vi "Config Alarm.vi"(0 "VISA resource name":refnum<visa-resource-name>, 1 "Alarm (F: Alarm Disabled)":bool, 2 "Beeper (F: Beeper Disabled)":bool, 3 "Latching (F: Alarm Latch OFF)":bool, 5 "Input (1)":dbl=1.0 min=1.0 max=8.0 step=1.0, 9 "Alarm Source (0:Kelvin)":u16(ring) items=["Kelvin", "Celsius", "Sensor Units", "Linear Data"], 11 "error in (no error)":errorcluster, 12 "High Value (0.0000)":dbl min=-9999.9 max=9999.9 step=0.0001 format="%.4f", 13 "Deadband (0.0000)":dbl min=0.0 max=9999.9 step=0.0001 format="%.4f", 14 "Low Value (0.0000)":dbl min=-9999.9 max=9999.9 step=0.0001 format="%.4f") -> (4 "VISA resource name out":refnum<visa-resource-name>, 15 "error out":errorcluster)   [LabVIEW 2012, in "Lake Shore Cryotronics 218.lvlib"]
doc: "This VI configures all alarm functions for the selected input. Alarm functions include source, on/off, high value, low value, deadband, and latching parameters. This VI also enables/disables the system beeper, this control applies to all inputs."
uses:
  <instrlib>/Lake Shore Cryotronics 218/Lake Shore Cryotronics 218.lvlib
panel:
  # "Alarm Enabled"
  # "Alarm Latch ON"
  # "Alarm Disabled"
  # "Alarm Latch OFF"
  # "Beeper Enabled"
  # "Beeper Disabled"
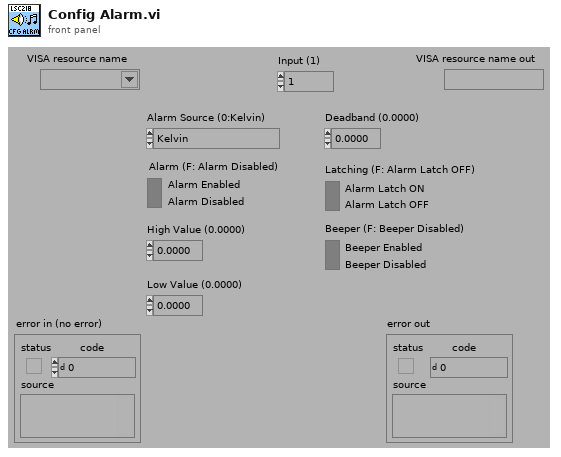
[diagram p1: front panel]
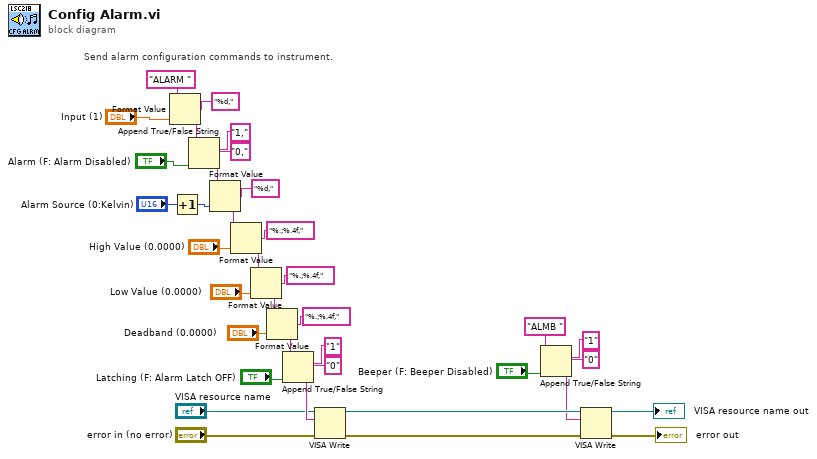
[diagram p0: block diagram]
diagram:
  # "Send alarm configuration commands to instrument."
  n1 = Format Value(string ("")="ALARM ", format string="%d,", value (0)="Input (1)") -> (output string=w21:string)
  n2 = Increment(x="Alarm Source (0:Kelvin)") -> (x+1=w23:u16)
  n3 = Append True/False String(1:"Alarm (F: Alarm Disabled)", 2:"0,", 3:"1,", 4:w21) -> (0:w20:string)
  n4 = Format Value(string ("")=w20, format string="%d,", value (0)=w23) -> (output string=w19:string)
  n5 = Format Value(string ("")=w19, format string="%.;%.4f,", value (0)="High Value (0.0000)") -> (output string=w18:string)
  n6 = Format Value(string ("")=w18, format string="%.;%.4f,", value (0)="Low Value (0.0000)") -> (output string=w16:string)
  n7 = Format Value(string ("")=w16, format string="%.;%.4f,", value (0)="Deadband (0.0000)") -> (output string=w11:string)
  n8 = Append True/False String(1:"Latching (F: Alarm Latch OFF)", 2:"0", 3:"1", 4:w11) -> (0:w10:string)
  n9 = VISA Write(VISA resource name="VISA resource name", write buffer=w10, error in (no error)="error in (no error)") -> (VISA resource name out=w32:refnum<visa-resource-name>, error out=w31:errorcluster)  [unwired: 1 out]
  n10 = Append True/False String(1:"Beeper (F: Beeper Disabled)", 2:"0", 3:"1", 4:"ALMB ") -> (0:w7:string)
  n11 = VISA Write(VISA resource name=w32, write buffer=w7, error in (no error)=w31) -> (VISA resource name out=→"VISA resource name out":refnum<visa-resource-name>, error out=→"error out":errorcluster)  [unwired: 1 out]
